vi "Accumulate and average data.vi"(7 "# Scans Accululated In":i32, 9 "Accumulated Array":dbl[](array[numeric]), 10 "Raw Data In":dbl[][](array[numeric])) -> (2 "# Scans Accumulated Out":i32, 3 "Accumulated Array Out":dbl[](array[numeric]))   [LabVIEW 2018]
doc: "Author: Scott Hannahs <sth@magnet.fsu.edu>\nCopyright 2018 Florida State University, All rights reserved."
uses:
  RT Host Globals.vi
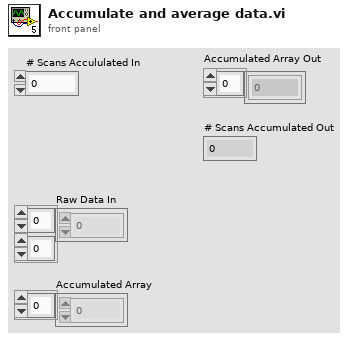
[diagram p1: front panel]
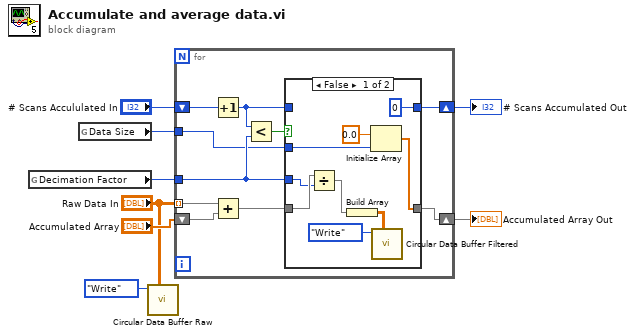
[diagram p0: block diagram]
diagram:
  n1 = global read "RT Host Globals.vi" "Decimation Factor"() -> (w4:u32)
  n2 = global read "RT Host Globals.vi" "Data Size"() -> (w3:u32)
  n3 = call "Circular Data Buffer Raw.vi"("Data In"="Raw Data In", "Enum"=enum16{"Initialize", "Write", "Read", "Clear"}."Write") -> ()  [unwired: 7 in, 3 out]
  n4 = for {
    shift-right: [w13] -> w8
    shift-left: "# Scans Accululated In" -> [w17]
    tunnel: "Raw Data In" -> [w15] mode=indexing
    shift-right: [w11] -> w6
    shift-left: "Accumulated Array" -> [w18]
    tunnel: w4 -> [w14]
    tunnel: w3 -> [w9]
    n5 = Increment(x=w17) -> (x+1=w12:i32)
    n6 = Add(x=w15, y=w18) -> (x+y=w10:dbl[])
    n7 = Less?(x=w12, y=w14) -> (x < y?=w16:bool)
    n8 = case shown="False" w16 {
      tunnel: w10 -> [w27 w28]
      tunnel: w14 -> [w26 _]
      tunnel: [0 w29] -> w13
      tunnel: w12 -> [_ w29]
      tunnel: [w23 w28] -> w11
      tunnel: w9 -> [w22 _]
      frame False {
        n9 = Divide(x=w27, y=w26) -> (x/y=w20:dbl[])
        n10 = Build Array(w20) -> (w19:dbl[][])
        n11 = Initialize Array(0.0, w22) -> (w23:dbl[])
        n12 = call "Circular Data Buffer Filtered.vi"("Data In"=w19, "Action"=enum16{"Initialize", "Write", "Read", "Clear"}."Write" ("Enum")) -> ()  [unwired: 7 in, 3 out]
      }
      frame True {
      }
    }
  }
  "# Scans Accumulated Out" <- w8
  "Accumulated Array Out" <- w6
